vi "Config1.vi"(1 "file path (dialog if empty)":path) -> (0 "Distancias":dbl[](array[numeric]))   [LabVIEW 2015]
panel:
  out "text":string
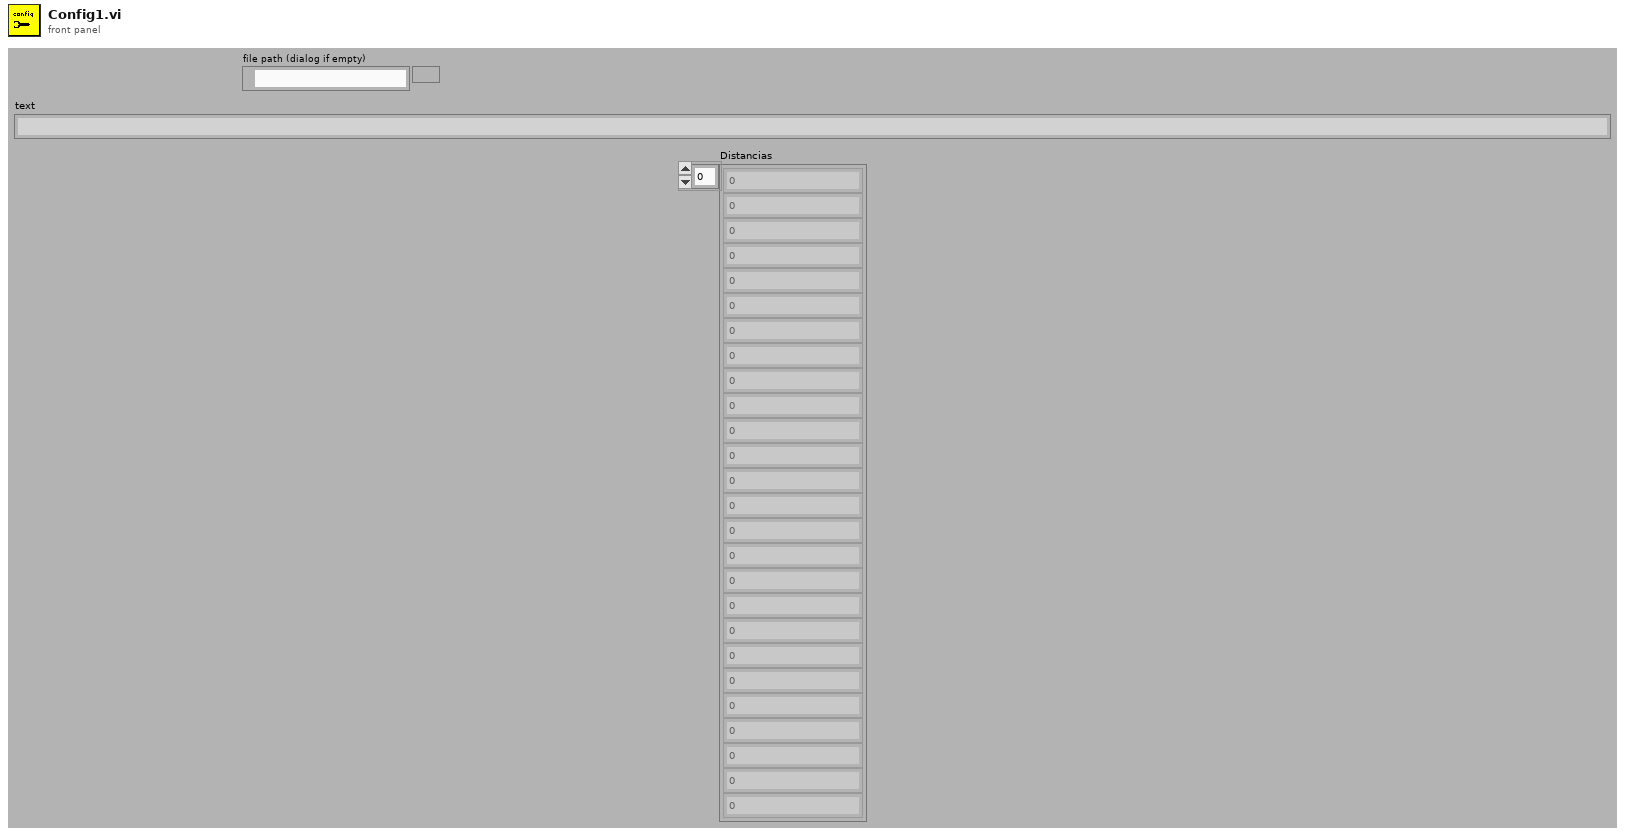
[diagram p1: front panel]
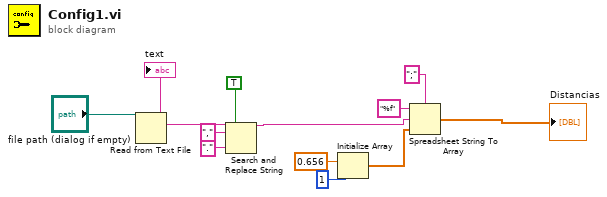
[diagram p0: block diagram]
diagram:
  n1 = Read from Text File(file (use dialog)="file path (dialog if empty)") -> (text=w5:string)  [unwired: 3 in, 3 out]
  "text" <- w5
  n2 = Search and Replace String(replace all?=TRUE ("replace all? (F)"), input string=w5, search string=",", replace string="." ("replace string (\"\")")) -> (result string=w4:string)  [unwired: 4 in, 3 out]
  n3 = Initialize Array(0.656 ("element"), 1 ("dimension size")) -> (w7:dbl[])
  n4 = Spreadsheet String To Array(delimiter (Tab)=";" ("prompt (Open existing file)"), format string="%f", spreadsheet string=w4, array type (2D Dbl)=w7) -> (array=→"Distancias":dbl[])
